vi "Mouse Compass Test.vi"() -> ()   [LabVIEW 2012]
uses:
  <vilib>/FPGAPlugInAG/sbRIO-9636/niLvFpga_Open_sbRIO-9636.vi
  <vilib>/rvi/interface/common/dynamic/niFpgaDynamicAddResources.vi
  <vilib>/FPGAPlugInAG/Dynamic/niLvFpga_Close_Dynamic.vi
  <vilib>/rvi/interface/nirviOpenFPGA/nirviOpenFPGA.xnode
  FPGA Bitfiles/NIARC_FPGATarget_FPGACompile_e4XhunWUay0.lvbitx
  <vilib>/rvi/interface/nirviCloseFPGA/nirviCloseFPGA.xnode
  Compass/Compass IO.lvlib
panel:
  out "Heading":dbl(graph)
  in  "Reset":bool
  out "Heading (deg)":dbl
  in  "stop":bool
  out "Waveform Chart":cluster{dbl, dbl}(graph)
  out "read buffer":string
  out "Full packet?":bool
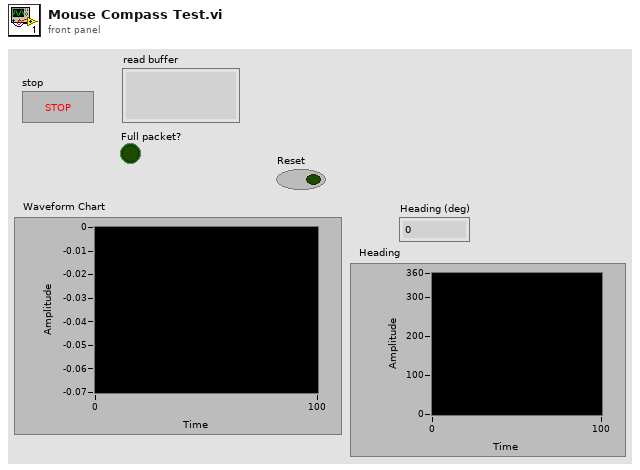
[diagram p1: front panel]
types:
  T1 = cluster{"FPGA VI Reference":refnum<k20>, "Port Number":u8}
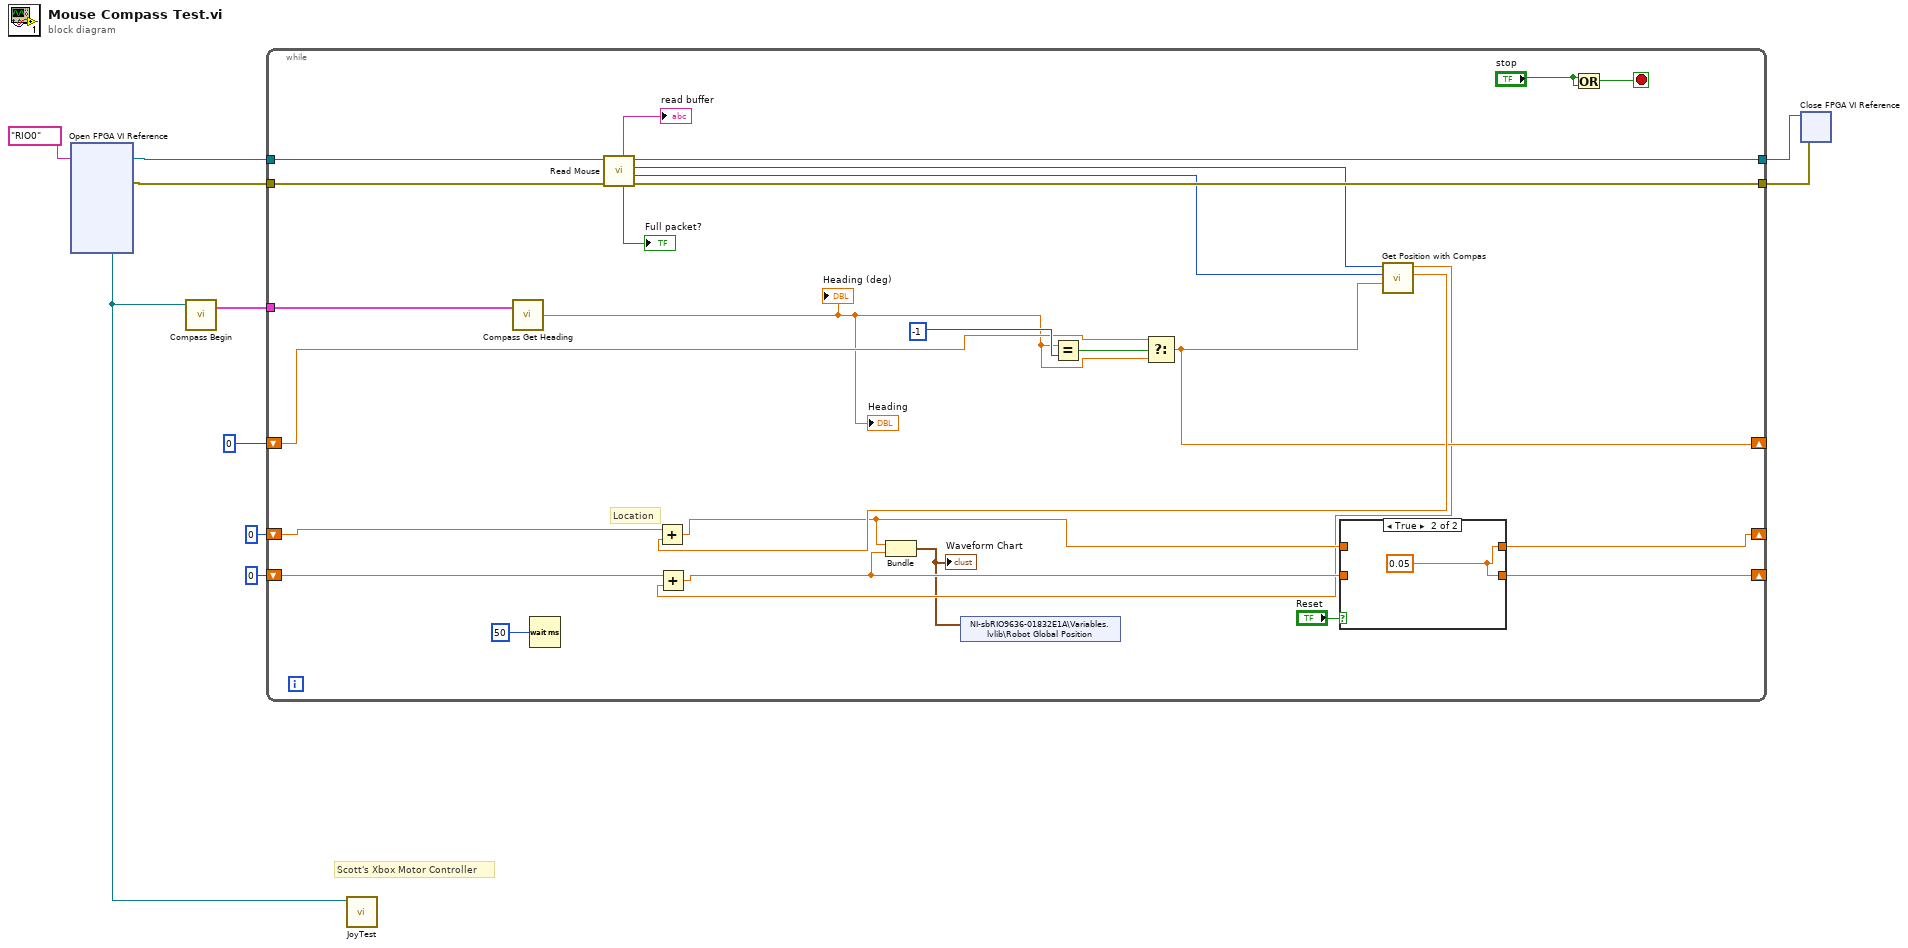
[diagram p0: block diagram]
diagram:
  # "Scott's Xbox Motor Controller"
  n1 = xnode "Open FPGA VI Reference"("resource name"=tag "RIO0") -> ("FPGA VI Reference Out"=w2:refnum<k20>, "error out"=w5:errorcluster)  [unwired: 1 in]
  n2 = call "Compass Begin.vi"("FPGA VI Reference"=w2) -> ("FPGA Information Out"=w4:T1)  [unwired: 3 in, 1 out]
  n3 = while {
    shift-right: [w26] -> _
    shift-left: 0 -> [w35]
    shift-right: [w25] -> _
    shift-left: 0 -> [w34]
    shift-right: [w27] -> _
    shift-left: i16 0 -> [w28]
    tunnel: [w32] -> w6
    tunnel: w5 -> [w23]
    tunnel: w4 -> [w22]
    tunnel: w2 -> [w21]
    tunnel: [w20] -> w3
    stop <- w33 stop-if-true
    # "Location"
    n4 = call "Compass Get Heading.vi"("FPGA Information In"=w22) -> ("Heading (deg)"=w14:dbl)  [unwired: 1 in, 2 out]
    "Heading (deg)" <- w14
    "Heading" <- w14
    n5 = Wait (ms)(milliseconds to wait=u32 50) -> ()  [unwired: 1 out]
    n6 = call "Read Mouse.vi"("error in (no error)"=w23, "Refnum in"=w21) -> ("error out"=w32:errorcluster, "Delta y"=w10:i16, "Delta x"=w12:i16, "Refnum out"=w20:refnum<k20>, "Full packet?"=→"Full packet?":bool, "read buffer"=→"read buffer":string)  [unwired: 4 in]
    n7 = Equal?(x=w14, y=i16 -1) -> (x = y?=w30:bool)
    n8 = Select(t=w28, s=w30, f=w14) -> (s? t:f=w27:dbl)
    n9 = call "Get Position with Compas.vi"("Heading (deg)"=w27, "Delta y"=w10, "Delta x"=w12) -> ("y out"=w31:dbl, "x out"=w17:dbl)  [unwired: 7 in]
    n10 = Add(x=w35, y=w31) -> (x+y=w19:dbl)
    n11 = Add(x=w34, y=w17) -> (x+y=w18:dbl)
    n12 = Bundle(w19, w18) -> (w15:cluster{dbl, dbl})  [unwired: 1 in]
    "Waveform Chart" <- w15
    n13 = shared-variable "NI-sbRIO9636-01832E1A\\Variables.lvlib\\Robot Global Position"(w15) -> ()  [unwired: 1 in, 1 out]
    n14 = case shown="True" "Reset" {
      tunnel: [w38 w39] -> w26
      tunnel: w19 -> [w38 _]
      tunnel: w18 -> [w37 _]
      tunnel: [w37 w39] -> w25
      frame False {
      }
      frame True {
        w39 = 0.05
      }
    }
    n15 = Or(x="stop", y="stop") -> (x .or. y?=w33:bool)
  }
  n16 = call "JoyTest.vi"("FPGA Reference In"=w2) -> ()  [unwired: 11 in]
  n17 = xnode "Close FPGA VI Reference"("FPGA VI Reference In"=w3, "error in"=w6) -> ()  [unwired: 1 out]
